vi "GetOwner.vi"(6 "error in":errorcluster, 9 "Control in":refnum<class "Control.lvclass">) -> (0 "error out":errorcluster, 3 "Control out":refnum<class "Control.lvclass">, 4 "Owner":i32)   [LabVIEW 2014, in "Raspberry Pi Compatible Compiler for LabVIEW.lvlib" / "Control.lvclass"]
uses:
  Control.lvclass
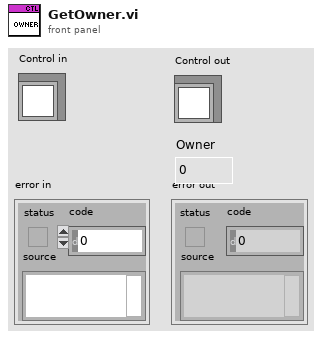
[diagram p1: front panel]
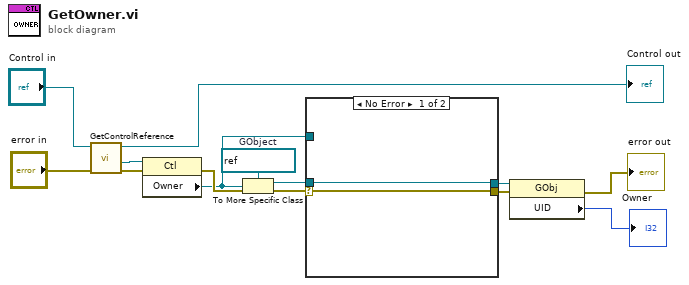
[diagram p0: block diagram]
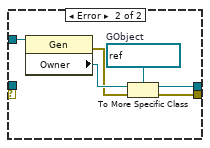
[diagram p2: hidden frame]
diagram:
  w5 = refnum<vi> refnum  # GObject
  n1 = call "GetControlReference.vi"("error in"="error in", "Control in"="Control in") -> ("error out"=w11:errorcluster, "control reference"=w12:refnum<vi>, "Control out"=→"Control out":refnum<class "Control.lvclass">)  [unwired: 7 in]
  n2 = property class="Ctl"(reference=w12, error in=w11) -> (error out=w4:errorcluster, "Owner"=w1:refnum<vi>)  [unwired: 1 out]
  n3 = To More Specific Class(target class=w5, reference=w1, error in=w4) -> (specific class reference=w2:refnum<vi>, error out=w3:errorcluster)
  n4 = case shown="No Error" w3 {
    selector: w3 -> [w15 _]
    tunnel: [w16 w22] -> w8
    tunnel: [w15 w21] -> w7
    tunnel: w2 -> [w16 _]
    tunnel: w1 -> [_ w19]
    frame No Error {
    }
    frame Error {
      w20 = refnum<vi> refnum  # GObject
      n5 = property class="Gen"(reference=w19) -> (error out=w17:errorcluster, "Owner"=w18:refnum<vi>)  [unwired: 1 in, 1 out]
      n6 = To More Specific Class(target class=w20, reference=w18, error in=w17) -> (specific class reference=w22:refnum<vi>, error out=w21:errorcluster)
    }
  }
  n7 = property class="GObj"(reference=w8, error in=w7) -> (error out=→"error out":errorcluster, "UID"=→"Owner":i32)  [unwired: 1 out]
